vi "rand out.vi"(7 "Min/Max":cluster{"Min":dbl, "Max":dbl}) -> (2 "rand out":dbl)   [LabVIEW 2015]
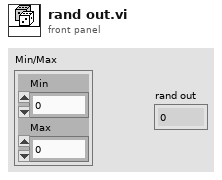
[diagram p1: front panel]
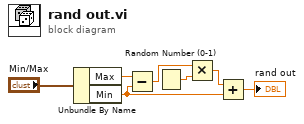
[diagram p0: block diagram]
diagram:
  n1 = Unbundle By Name("Min/Max") -> ("Max"=w6:dbl, "Min"=w2:dbl)
  n2 = Subtract(x=w6, y=w2) -> (x-y=w5:dbl)
  n3 = Random Number (0-1)() -> (number: 0 to 1=w4:dbl)
  n4 = Multiply(x=w5, y=w4) -> (x*y=w3:dbl)
  n5 = Add(x=w3, y=w2) -> (x+y=→"rand out":dbl)
